vi "example.vi"() -> ()   [LabVIEW 2016]
panel:
  out "TimestampArray":u64[](array[numeric])
  out "timestamp":timestamp
  out "waveformDbl":waveform(dbl)
  out "Some Indicator 2":i32
  out "arrayDbl":dbl[](array[numeric]) caption="arrayDble"
  out "Some Indicator":i32
  out "some_struct":cluster{"t0":timestamp, "dt":dbl, "Y":dbl[]}
  in  "Some Bool":bool
  out "arrayU16":u16[](array[numeric])
  in  "Some String":string
  in  "Some Control":dbl
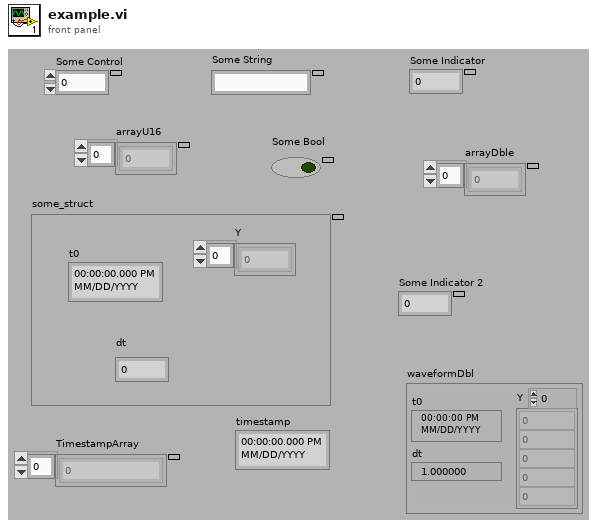
[diagram p1: front panel]
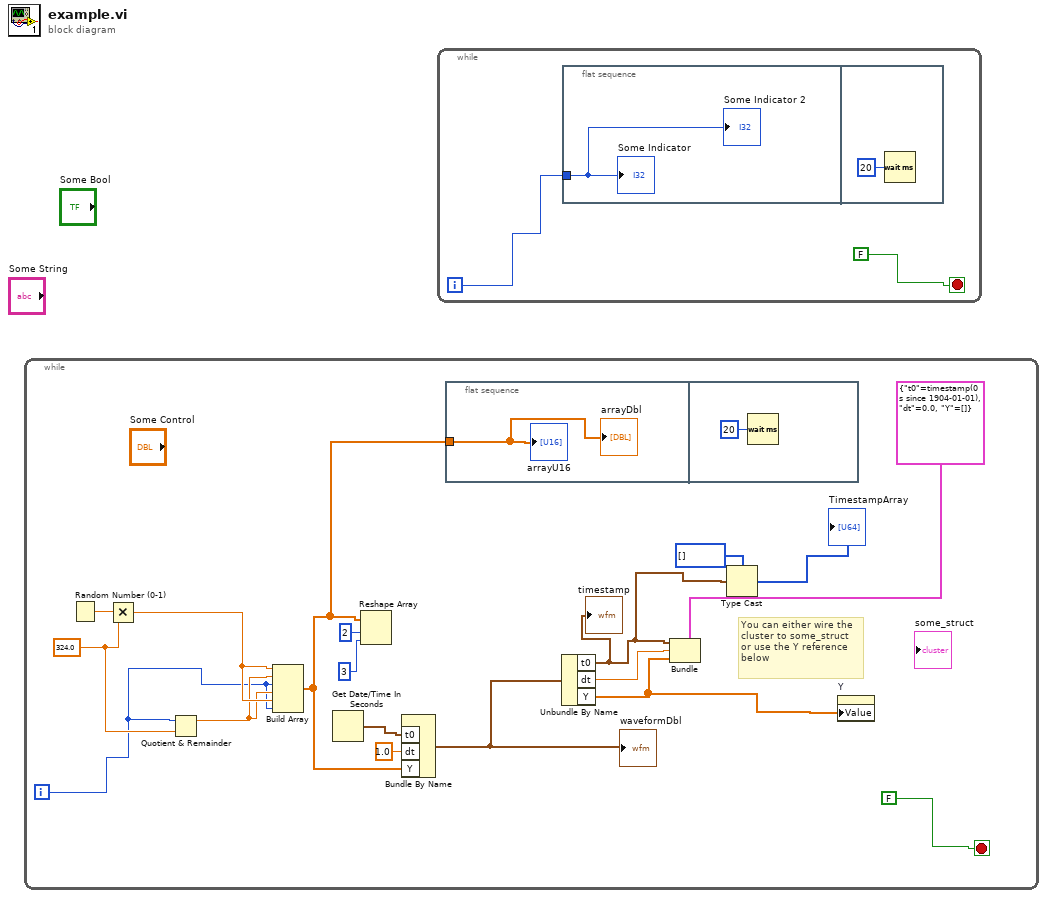
[diagram p0: block diagram]
diagram:
  n1 = while {
    i -> [w11]
    stop <- FALSE ("Some Button") stop-if-true
    w12 = 324.0 ("y")
    # "You can either wire the\ncluster to some_struct\nor use the Y reference \nbelow"
    n2 = Random Number (0-1)() -> (number: 0 to 1=w15:dbl)
    n3 = Multiply(x=w15, y=w12) -> (x*y=w14:dbl)
    n4 = Quotient & Remainder(x=w11, y=w12) -> (x-y*floor(x/y)=w13:dbl)  [unwired: 1 out]
    n5 = Build Array(w14, w13, w11, w13, w14, w11) -> (w6:dbl[])
    n6 = Get Date/Time In Seconds() -> (seconds since 1Jan1904=w9:timestamp)
    n7 = Reshape Array(w6, 2 ("dimension size"), 3 ("dimension size")) -> ()  [unwired: 1 out]
    n8 = Bundle By Name("t0"=w9, "dt"=1.0, "Y"=w6) -> (w5:waveform(dbl))  [unwired: 1 in]
    "waveformDbl" <- w5
    n9 = flat-sequence {
      tunnel: w6 -> [w19]
      frame #0 {
        "arrayU16" <- w19
        "arrayDbl" <- w19
      }
      frame #1 {
        n10 = Wait (ms)(milliseconds to wait=u32 20) -> ()  [unwired: 1 out]
      }
    }
    n11 = Unbundle By Name(w5) -> ("t0"=w4:timestamp, "dt"=w7:dbl, "Y"=w1:dbl[])
    "timestamp" <- w4
    n12 = Bundle(cluster=cluster{"t0":timestamp, "dt":dbl, "Y":dbl[]} {"t0"=timestamp(0 s since 1904-01-01), "dt"=0.0, "Y"=[]} ("Cluster"), "t0"=w4, "dt"=w7, "Y"=w1) -> ()  [unwired: 1 out]
    n13 = Type Cast(type=u64[] [] ("Array"), x=w4) -> (*(type *) &x=→"TimestampArray":u64[])
    n14 = property on="Y" class="Arr (strict)"("Value"=w1) -> ()  [unwired: 2 in, 2 out]
  }
  n15 = while {
    i -> [w21]
    stop <- FALSE ("Some Button") stop-if-true
    n16 = flat-sequence {
      tunnel: w21 -> [w23]
      frame #0 {
        "Some Indicator" <- w23
        "Some Indicator 2" <- w23
      }
      frame #1 {
        n17 = Wait (ms)(milliseconds to wait=u32 20) -> ()  [unwired: 1 out]
      }
    }
  }
